vi "Read Py File Path.vi"(8 "error in (no error)":errorcluster, 11 "Py Doc in":refnum<class "Py Doc.lvclass">) -> (0 "error out":errorcluster, 2 "Py File Path":path, 3 "Py Doc out":refnum<class "Py Doc.lvclass">)   [LabVIEW 2016, in "Py Doc.lvclass"]
uses:
  Py Doc.lvclass
  Py Doc.lvclass/Py Doc.ctl
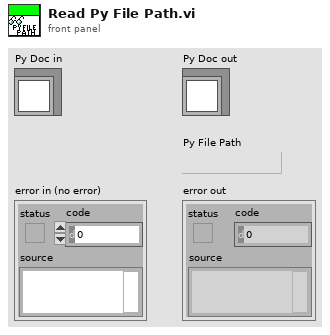
[diagram p1: front panel]
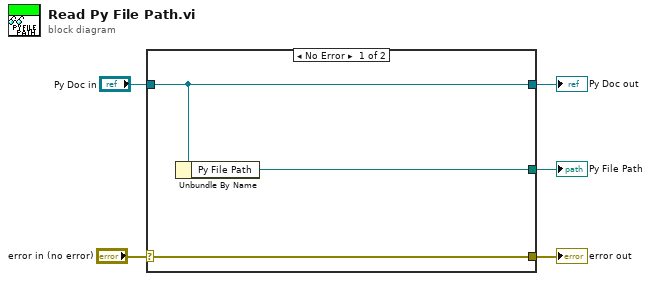
[diagram p0: block diagram]
diagram:
  n1 = case shown="No Error" "error in (no error)" {
    selector: "error in (no error)" -> [w8 w9]
    tunnel: [w8 w9] -> w4
    tunnel: [w7 w10] -> w2
    tunnel: "Py Doc in" -> [w7 w10]
    tunnel: [w6 _] -> w1
    frame No Error {
      n2 = Unbundle By Name(w7) -> ("Py File Path"=w6:path)
    }
    frame Error {
    }
  }
  "error out" <- w4
  "Py Doc out" <- w2
  "Py File Path" <- w1
